vi "TestOrientationStateMachine.vi"() -> ()   [LabVIEW 2017]
uses:
  Controls/OrientationState.ctl
  Controls/RubikMoves.ctl
panel:
  out "Final Orientation":T1
  in  "Rubik's Moves":T2
  in  "Initial Orientation":T1
  # "Test without Hardware"
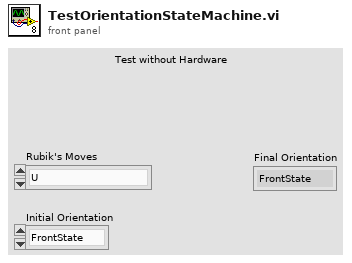
[diagram p1: front panel]
types:
  T1 = typedef "OrientationState.ctl" = enum16{"FrontState", "UpState", "BackState", "DownState"}
  T2 = typedef "RubikMoves.ctl" = enum16{"U", "U'", "F", "F'", "D", "D'", "B", "B'", "L", "L'", "R", "R'"}
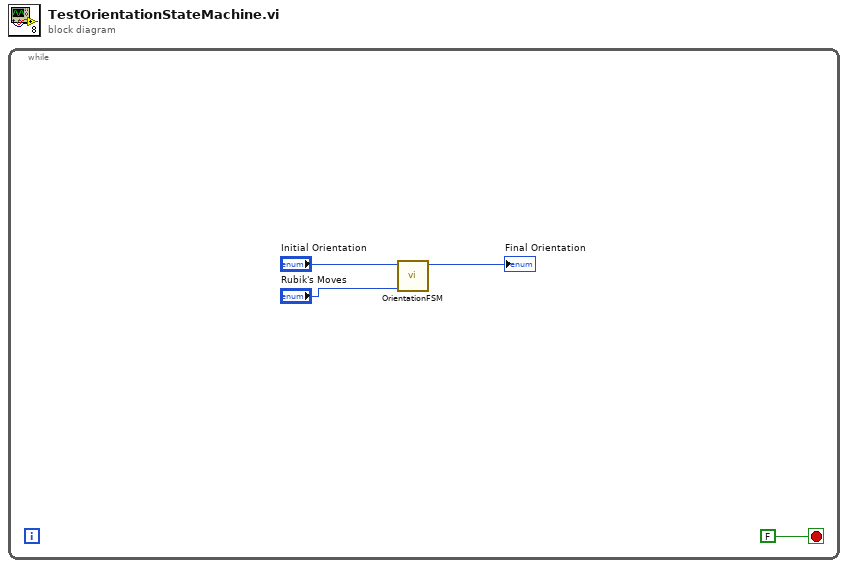
[diagram p0: block diagram]
diagram:
  n1 = while {
    stop <- FALSE stop-if-true
    n2 = call "OrientationFSM.vi"("Rubik's Moves"="Rubik's Moves", "Initial Orientation"="Initial Orientation") -> ("Final Orientation"=→"Final Orientation":T1)  [unwired: 9 in]
  }
